vi "Select Enabled Channel Coefficients.vi"(0 "configured scaling coefficients":T1[](array[typedef]), 5 "selected acq channels to store":bool[](array[boolean]), 7 "number of selected acq channels to store":u8) -> (4 "stored scaling coefficients":T1[](array[typedef]))   [LabVIEW 2021, in "Device Session.lvclass"]
doc: "Selects the scaling coefficients according to the number of channels enabled for acquisition.\n\n<B>Input Parameters</B>\n\n<B>configured scaling coefficients</B> specifies the scaling coefficients to select from.\n\n<B>selected acq channels to store</B> specifies the channels enabled for acquisition. Each element in this array is corresponds to a channel.\n\n<B>number of selected acq channels to store</B> specifies the number of enabled channels to store scaling coefficients for.\n\n<B>Output Parameters</B>\n\n<B>stored scaling coefficients</B> returns the scaling coefficients from the specified channels."
uses:
  Device Session.lvclass
  <instrlib>/_niInstr/Multirecord Acquisition/Interface/v1/Host/Public/Scaling Coefficient.ctl
  <instrlib>/_niInstr/Multirecord Acquisition/Interface/v1/Host/niInstr Multirecord Acquisition v1 Host.lvclass
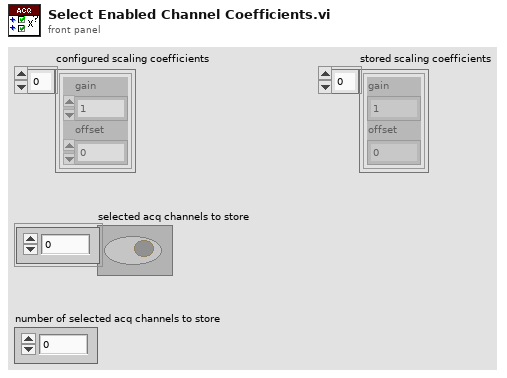
[diagram p1: front panel]
types:
  T1 = typedef "niInstr Multirecord Acquisition v1 Host.lvclass/Scaling Coefficient.ctl" = cluster{"gain":dbl, "offset":dbl}
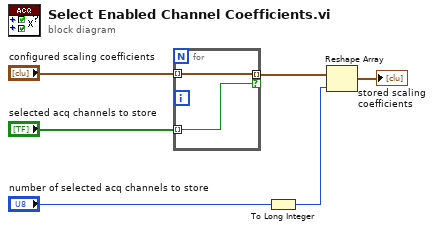
[diagram p0: block diagram]
diagram:
  n1 = for {
    tunnel: "selected acq channels to store" -> [w8] mode=indexing
    tunnel: [w7] -> w3 mode=indexing if=w8
    tunnel: "configured scaling coefficients" -> [w7] mode=indexing
  }
  n2 = To Long Integer(number="number of selected acq channels to store") -> (32bit integer=w5:i32)
  n3 = Reshape Array(w3, w5) -> (→"stored scaling coefficients":T1[])
